vi "Teleop.vi"(10 "Match Info":T1={"Autonomous Elapsed Seconds"=0.0, "TeleOp Elapsed Seconds"=0.0, "Disabled Elapsed Seconds"=0.0, "Visited Autonomous"=FALSE, "Visited TeleOp"=FALSE, "Visited Disabled"=FALSE, "Autonomous Settings"={"Autonomous Style"=enum."Independent", "VI Refnum"=refnum}}, 11 "Call Context":T2) -> ()   [LabVIEW 2011]
doc: "This VI is called for each TeleOp packet received from the DS where the robot is not disabled. It is often used to read from the joysticks and update I/O or to update setpoints for timed control loops. It should complete and return within 20 milliseconds or it may miss DS packets."
uses:
  <vilib>/Rock Robotics/WPI/DriverStation/WPI_DriverStationDerivedRobotMode.ctl
  <vilib>/Rock Robotics/WPI/DriverStation/WPI_DriverStationMatch Info.ctl
  Robot Global Data.vi
  System Set Points and States.vi
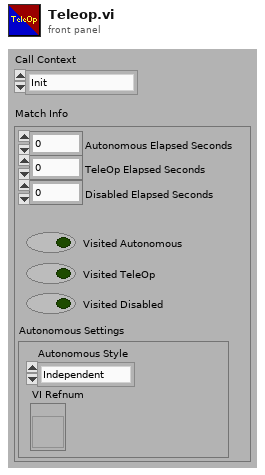
[diagram p1: front panel]
types:
  T1 = typedef "WPI_DriverStationMatch Info.ctl" = cluster{"Autonomous Elapsed Seconds":dbl, "TeleOp Elapsed Seconds":dbl, "Disabled Elapsed Seconds":dbl, "Visited Autonomous":bool, "Visited TeleOp":bool, "Visited Disabled":bool, "Autonomous Settings":cluster{"Autonomous Style":enum16{"Iterative", "Independent"}, "VI Refnum":refnum<vi>}}
  T2 = typedef "WPI_DriverStationDerivedRobotMode.ctl" = enum16{"Init", "Execute", "Stop"}
  T3 = typedef "WPI_JoystickDevRef.ctl" = cluster{"Device":T4}
  T4 = typedef "WPI_JoystickDeviceEnum.ctl" = enum16{"USB 1", "USB 2", "USB 3", "USB 4", "Kinect 1", "Kinect 2"}
  T5 = typedef "WPI_JoystickButtonState.ctl" = cluster{"Button 1":bool, "Button 2":bool, "Button 3":bool, "Button 4":bool, "Button 5":bool, "Button 6":bool, "Button 7":bool, "Button 8":bool, "Button 9":bool, "Button 10":bool, "Button 11":bool, "Button 12":bool}
  T6 = cluster{"axis 1 (x)":dbl, "axis 2 (y)":dbl, "axis 3 (throttle)":dbl, "axis 4":dbl, "axis 5":dbl, "axis 6":dbl}
  T7 = typedef "WPI_DigitalInputDevRef.ctl" = cluster{"DevStatus":errorcluster, "DIO Channel":T8, "Digital Module":T9}
  T8 = typedef "FPGA_DIOChannel.ctl" = enum8{"DIO 1", "DIO 2", "DIO 3", "DIO 4", "DIO 5", "DIO 6", "DIO 7", "DIO 8", "DIO 9", "DIO 10", "DIO 11", "DIO 12", "DIO 13", "DIO 14", "Invalid"}
  T9 = typedef "FPGA_TypedefDigitalModule.ctl" = enum16{"Digital Module 1", "Digital Module 2"}
  T10 = typedef "WPI_RobotDriveDevRef.ctl" = cluster{"DevStatus":errorcluster, "Motors[]":T11[], "Square Inputs":bool, "Max Output":dbl, "Isochronous":bool}
  T11 = typedef "WPI_MotorControlDeviceRef.ctl" = cluster{"DeviceStatus":errorcluster, "Type":enum16{"PWM", "CAN"}, "PWM":cluster{"Digital Module":T9, "PWM Channel":T12, "DeadBand":T13}, "CAN":cluster{"Device Number":u8, "Control Mode":T14, "Semaphore":T15, "Max Vout":dbl}, "Invert":bool, "TransformRef":T16, "InvTransformRef":T16}
  T12 = typedef "FPGA_DIOPWMChannel.ctl" = enum8{"PWM 1", "PWM 2", "PWM 3", "PWM 4", "PWM 5", "PWM 6", "PWM 7", "PWM 8", "PWM 9", "PWM 10", "Invalid"}
  T13 = typedef "WPI_PWMDeadband.ctl" = cluster{"Name":string, "maxPositivePwm":i32, "minPositivePwm":i32, "centerPwm":i32, "maxNegativePwm":i32, "minNegativePwm":i32, "angularRange":u16}
  T14 = typedef "WPI_CANJaguar_ControlMode.ctl" = enum8{"Percent VBus", "Current", "Speed", "Position", "Voltage"}
  T15 = typedef "Semaphore RefNum" = refnum<k1>
  T16 = typedef "WPI_PWMTransform_ConPane.ctl" = refnum<vi>
  T17 = typedef "WPI_AnalogChannelDevRef.ctl" = cluster{"DevStatus":errorcluster, "Analog Module":T18, "Analog Channel":T19}
  T18 = typedef "FPGA_TypedefAnalogModule.ctl" = enum16{"Analog Module 1", "Analog Module 2"}
  T19 = typedef "FPGA_AIChannel.ctl" = enum8{"AI 1", "AI 2", "AI 3", "AI 4", "AI 5", "AI 6", "AI 7", "AI 8", "Invalid"}
  T20 = cluster{"Position":cluster{"X":dbl, "Y":dbl}, "Distance (ft)":dbl}[]
  T21 = cluster{"Target Info[0]":cluster{"Position":cluster{"X":dbl, "Y":dbl}, "Distance (ft)":dbl}, "Target Info[1]":cluster{"Position":cluster{"X":dbl, "Y":dbl}, "Distance (ft)":dbl}, "Target Info[2]":cluster{"Position":cluster{"X":dbl, "Y":dbl}, "Distance (ft)":dbl}, "Target Info[3]":cluster{"Position":cluster{"X":dbl, "Y":dbl}, "Distance (ft)":dbl}, "Target Info[4]":cluster{"Position":cluster{"X":dbl, "Y":dbl}, "Distance (ft)":dbl}, "Target Info[5]":cluster{"Position":cluster{"X":dbl, "Y":dbl}, "Distance (ft)":dbl}, "Target Info[6]":cluster{"Position":cluster{"X":dbl, "Y":dbl}, "Distance (ft)":dbl}, "Target Info[7]":cluster{"Position":cluster{"X":dbl, "Y":dbl}, "Distance (ft)":dbl}, "Target Info[8]":cluster{"Position":cluster{"X":dbl, "Y":dbl}, "Distance (ft)":dbl}}
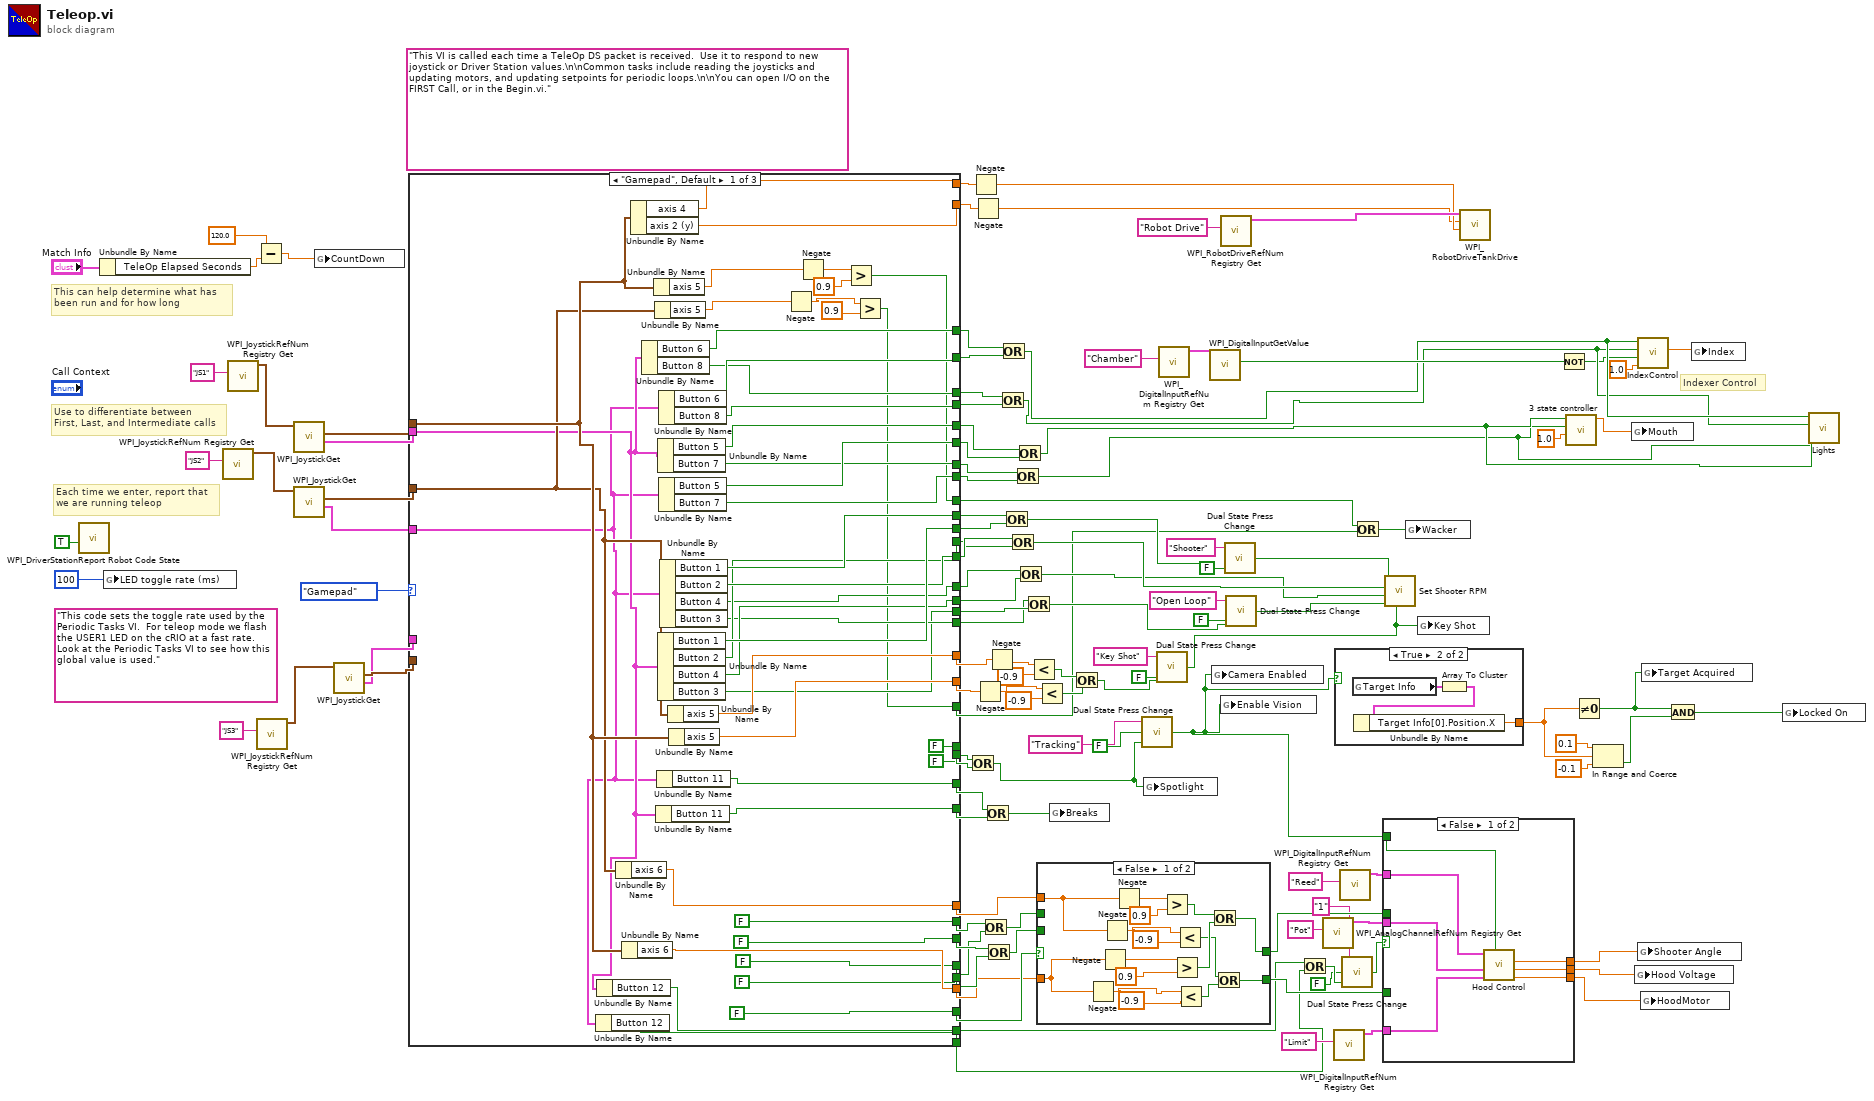
[diagram p0: block diagram]
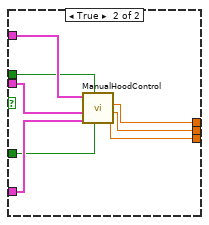
[diagram p2: hidden frame]
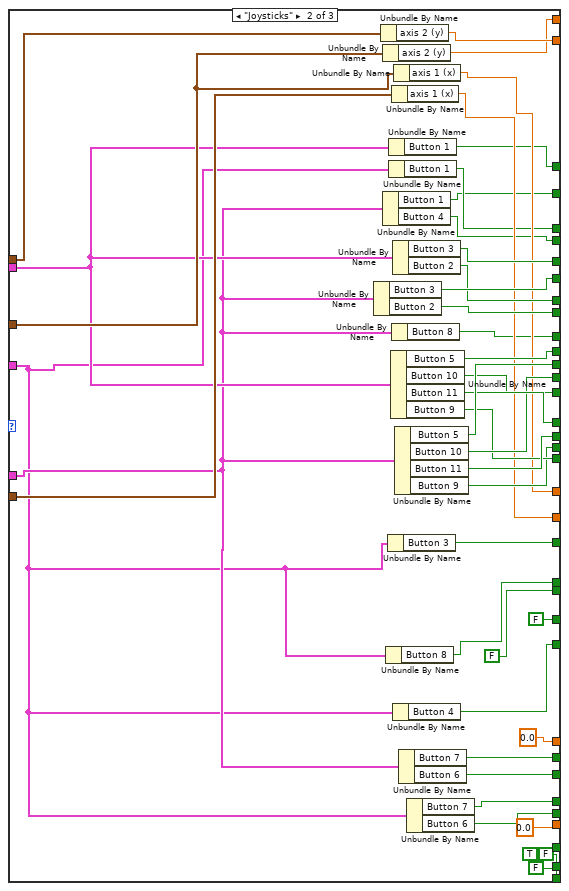
[diagram p4: hidden frame]
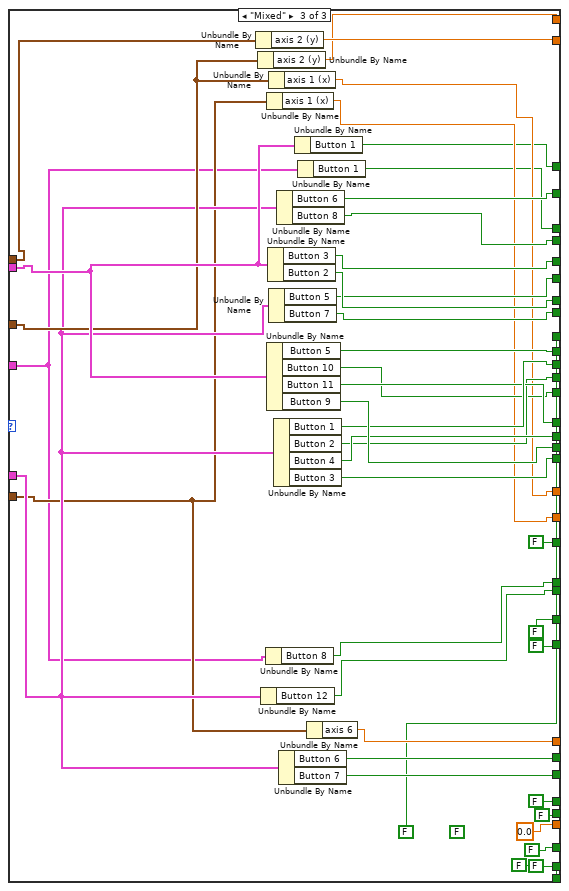
[diagram p5: hidden frame]
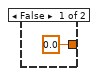
[diagram p6: hidden frame]
diagram:
  (unwired) "This code sets the toggle rate used by the Periodic Tasks VI.  For teleop mode we flash the USER1 LED on the cRIO at a fast rate.  Look at the Periodic Tasks VI to see how this global value is used."
  (unwired) "This VI is called each time a TeleOp DS packet is received.  Use it to respond to new joystick or Driver Station values.\n\nCommon tasks include reading the joysticks and updating motors, and updating setpoints for periodic loops.\n\nYou can open I/O on the FIRST Call, or in the Begin.vi."
  # "Indexer Control"
  # "Each time we enter, report that\nwe are running teleop"
  # "Use to differentiate between\nFirst, Last, and Intermediate calls"
  # "This can help determine what has\nbeen run and for how long"
  n1 = call <vilib>:"WPI_DriverStationReport Robot Code State.vi"("TeleOp"=TRUE ("Autonomous")) -> ()  [unwired: 10 in, 1 out]
  n2 = Unbundle By Name("Match Info") -> ("TeleOp Elapsed Seconds"=w94:dbl)
  n3 = global write "Robot Global Data.vi" "LED toggle rate (ms)"(u32 100 ("LED ms toggle rate")) -> ()
  n4 = call <vilib>:"WPI_JoystickRefNum Registry Get.vi"("refnum name"="JS2") -> ("JoystickDevRef"=w88:T3)  [unwired: 9 in, 1 out]
  n5 = call <vilib>:"WPI_JoystickRefNum Registry Get.vi"("refnum name"="JS1") -> ("JoystickDevRef"=w115:T3)  [unwired: 9 in, 1 out]
  n6 = Subtract(x=120.0, y=w94) -> (x-y=w60:dbl)
  n7 = call <vilib>:"WPI_JoystickRefNum Registry Get.vi"("refnum name"="JS3") -> ("JoystickDevRef"=w56:T3)  [unwired: 9 in, 1 out]
  n8 = call <vilib>:"WPI_JoystickGet.vi"("JoystickDevRef"=w115) -> ("Buttons"=w102:T5, "Axes"=w61:T6)  [unwired: 4 in, 1 out]
  n9 = call <vilib>:"WPI_JoystickGet.vi"("JoystickDevRef"=w88) -> ("Buttons"=w68:T5, "Axes"=w62:T6)  [unwired: 4 in, 1 out]
  n10 = global write "System Set Points and States.vi" "CountDown"(w60) -> ()
  n11 = call <vilib>:"WPI_JoystickGet.vi"("JoystickDevRef"=w56) -> ("Buttons"=w58:T5, "Axes"=w59:T6)  [unwired: 4 in, 1 out]
  n12 = case shown="\"Gamepad\", Default" enum16{"Gamepad", "Mixed", "Joysticks"}."Gamepad" {
    tunnel: [w164 w180 w217] -> w112
    tunnel: [w163 w181 w218] -> w111
    tunnel: w102 -> [w123 w179 w245]
    tunnel: [w162 0.0 ("axis 6") 0.0 ("axis 6")] -> w7
    tunnel: [w161 w198 w237] -> w87
    tunnel: [w160 w199 w236] -> w86
    tunnel: [w159 w196 w232] -> w84
    tunnel: [w158 w195 w233] -> w83
    tunnel: [w157 w194 w234] -> w81
    tunnel: [w156 w197 w235] -> w80
    tunnel: [w138 w192 w238] -> w78
    tunnel: [w155 w193 w239] -> w77
    tunnel: [w154 w175 w226] -> w75
    tunnel: [w153 w178 w215] -> w74
    tunnel: [w152 w177 w214] -> w72
    tunnel: [w151 w174 w227] -> w71
    tunnel: [w150 w191 w228] -> w69
    tunnel: w68 -> [w122 w169 w216]
    tunnel: [w141 w189 w230] -> w40
    tunnel: [w142 w190 w229] -> w41
    tunnel: [w149 w188 w231] -> w66
    tunnel: [FALSE ("Button 8") w200 w240] -> w64
    tunnel: [FALSE ("Button 12") FALSE ("Button 12") w222] -> w63
    tunnel: [w148 0.0 ("axis 6") w219] -> w8
    tunnel: w62 -> [w136 w182 w223]
    tunnel: w61 -> [w137 w204 w246]
    tunnel: w59 -> [_ w205 w220]
    tunnel: w58 -> [_ w173 w221]
    tunnel: [w146 w187 w225] -> w49
    tunnel: [w147 w186 w224] -> w48
    tunnel: [FALSE ("Button 6") w185 w242] -> w25
    tunnel: [FALSE ("Button 7") w184 w241] -> w29
    tunnel: [FALSE TRUE FALSE] -> w47
    tunnel: [w129 w176 FALSE ("Button 1")] -> w31
    tunnel: [w128 w172 FALSE ("Button 3")] -> w32
    tunnel: [FALSE ("Button 7") w171 FALSE ("Button 7")] -> w28
    tunnel: [FALSE ("Button 6") w170 FALSE ("Button 6")] -> w26
    tunnel: [w125 FALSE ("Button 12") FALSE ("Button 4")] -> w19
    tunnel: [w124 w168 FALSE ("Button 4")] -> w18
    tunnel: [w121 FALSE ("Button 11") FALSE ("Button 11")] -> w2
    tunnel: [w120 FALSE ("Button 11") FALSE ("Button 11")] -> w1
    frame "Gamepad", Default {
      n13 = Unbundle By Name(w122) -> ("Button 12"=w120:bool)
      n14 = Unbundle By Name(w123) -> ("Button 12"=w121:bool)
      n15 = Unbundle By Name(w136) -> ("axis 6"=w148:dbl)
      n16 = Unbundle By Name(w137) -> ("axis 6"=w162:dbl)
      n17 = Unbundle By Name(w137) -> ("axis 4"=w164:dbl, "axis 2 (y)"=w163:dbl)
      n18 = Unbundle By Name(w123) -> ("Button 6"=w153:bool, "Button 8"=w152:bool)
      n19 = Unbundle By Name(w137) -> ("axis 5"=w135:dbl)
      n20 = Unbundle By Name(w136) -> ("axis 5"=w134:dbl)
      n21 = Unbundle By Name(w123) -> ("Button 11"=w124:bool)
      n22 = Unbundle By Name(w122) -> ("Button 11"=w125:bool)
      n23 = Unbundle By Name(w123) -> ("Button 5"=w150:bool, "Button 7"=w141:bool)
      n24 = Unbundle By Name(w123) -> ("Button 1"=w160:bool, "Button 2"=w158:bool, "Button 4"=w157:bool, "Button 3"=w138:bool)
      n25 = Unbundle By Name(w122) -> ("Button 6"=w154:bool, "Button 8"=w151:bool)
      n26 = Unbundle By Name(w122) -> ("Button 5"=w142:bool, "Button 7"=w149:bool)
      n27 = Unbundle By Name(w122) -> ("Button 1"=w161:bool, "Button 2"=w159:bool, "Button 4"=w156:bool, "Button 3"=w155:bool)
      n28 = Unbundle By Name(w136) -> ("axis 5"=w147:dbl)
      n29 = Unbundle By Name(w137) -> ("axis 5"=w146:dbl)
      n30 = Negate(x=w134) -> (-x=w131:dbl)
      n31 = Negate(x=w135) -> (-x=w133:dbl)
      n32 = Greater?(x=w133, y=0.9) -> (0:w129:bool)
      n33 = Greater?(x=w131, y=0.9) -> (0:w128:bool)
    }
    frame "Joysticks" {
      n34 = Unbundle By Name(w173) -> ("Button 3"=w190:bool, "Button 2"=w188:bool)
      n35 = Unbundle By Name(w204) -> ("axis 2 (y)"=w181:dbl)
      n36 = Unbundle By Name(w182) -> ("axis 2 (y)"=w180:dbl)
      n37 = Unbundle By Name(w173) -> ("Button 1"=w175:bool, "Button 4"=w174:bool)
      n38 = Unbundle By Name(w169) -> ("Button 8"=w200:bool)
      n39 = Unbundle By Name(w169) -> ("Button 3"=w172:bool)
      n40 = Unbundle By Name(w179) -> ("Button 1"=w178:bool)
      n41 = Unbundle By Name(w169) -> ("Button 1"=w177:bool)
      n42 = Unbundle By Name(w179) -> ("Button 5"=w198:bool, "Button 10"=w196:bool, "Button 11"=w197:bool, "Button 9"=w193:bool)
      n43 = Unbundle By Name(w205) -> ("axis 1 (x)"=w187:dbl)
      n44 = Unbundle By Name(w173) -> ("Button 8"=w176:bool)
      n45 = Unbundle By Name(w179) -> ("Button 3"=w191:bool, "Button 2"=w189:bool)
      n46 = Unbundle By Name(w169) -> ("Button 4"=w168:bool)
      n47 = Unbundle By Name(w182) -> ("axis 1 (x)"=w186:dbl)
      n48 = Unbundle By Name(w173) -> ("Button 5"=w199:bool, "Button 10"=w195:bool, "Button 11"=w194:bool, "Button 9"=w192:bool)
      n49 = Unbundle By Name(w173) -> ("Button 7"=w185:bool, "Button 6"=w184:bool)
      n50 = Unbundle By Name(w169) -> ("Button 7"=w170:bool, "Button 6"=w171:bool)
    }
    frame "Mixed" {
      (unwired) FALSE ("Button 4")
      n51 = Unbundle By Name(w246) -> ("axis 2 (y)"=w218:dbl)
      n52 = Unbundle By Name(w223) -> ("axis 2 (y)"=w217:dbl)
      n53 = Unbundle By Name(w221) -> ("Button 12"=w222:bool)
      n54 = Unbundle By Name(w216) -> ("Button 8"=w240:bool)
      n55 = Unbundle By Name(w220) -> ("axis 1 (x)"=w225:dbl)
      n56 = Unbundle By Name(w245) -> ("Button 5"=w237:bool, "Button 10"=w232:bool, "Button 11"=w235:bool, "Button 9"=w238:bool)
      n57 = Unbundle By Name(w245) -> ("Button 3"=w228:bool, "Button 2"=w230:bool)
      n58 = Unbundle By Name(w223) -> ("axis 1 (x)"=w224:dbl)
      n59 = Unbundle By Name(w221) -> ("Button 5"=w229:bool, "Button 7"=w231:bool)
      n60 = Unbundle By Name(w221) -> ("Button 1"=w236:bool, "Button 2"=w233:bool, "Button 4"=w234:bool, "Button 3"=w239:bool)
      n61 = Unbundle By Name(w221) -> ("Button 6"=w226:bool, "Button 8"=w227:bool)
      n62 = Unbundle By Name(w221) -> ("Button 6"=w242:bool, "Button 7"=w241:bool)
      n63 = Unbundle By Name(w245) -> ("Button 1"=w215:bool)
      n64 = Unbundle By Name(w216) -> ("Button 1"=w214:bool)
      n65 = Unbundle By Name(w220) -> ("axis 6"=w219:dbl)
    }
  }
  n66 = Or(x=w64, y=w63) -> (x .or. y?=w37:bool)
  n67 = Negate(x=w112) -> (-x=w43:dbl)
  n68 = Negate(x=w111) -> (-x=w42:dbl)
  n69 = Negate(x=w49) -> (-x=w52:dbl)
  n70 = Or(x=w25, y=w26) -> (x .or. y?=w27:bool)
  n71 = Or(x=w19, y=w18) -> (x .or. y?=w20:bool)
  n72 = Or(x=w29, y=w28) -> (x .or. y?=w30:bool)
  n73 = Negate(x=w48) -> (-x=w54:dbl)
  n74 = Or(x=w72, y=w71) -> (x .or. y?=w70:bool)
  n75 = Or(x=w74, y=w75) -> (x .or. y?=w73:bool)
  n76 = Or(x=w87, y=w86) -> (x .or. y?=w85:bool)
  n77 = Or(x=w84, y=w83) -> (x .or. y?=w82:bool)
  n78 = Or(x=w40, y=w66) -> (x .or. y?=w65:bool)
  n79 = Or(x=w69, y=w41) -> (x .or. y?=w67:bool)
  n80 = Or(x=w80, y=w81) -> (x .or. y?=w79:bool)
  n81 = Or(x=w77, y=w78) -> (x .or. y?=w76:bool)
  n82 = Less?(x=w54, y=-0.9) -> (x < y?=w51:bool)
  n83 = Less?(x=w52, y=-0.9) -> (x < y?=w50:bool)
  n84 = case shown="False" w47 {
    tunnel: w7 -> [w253 _]
    tunnel: w8 -> [w254 _]
    tunnel: [w250 w263] -> w10
    tunnel: [w247 w264] -> w9
    tunnel: w27 -> [_ w264]
    tunnel: w30 -> [_ w263]
    frame False {
      n85 = Negate(x=w253) -> (-x=w258:dbl)
      n86 = Negate(x=w253) -> (-x=w260:dbl)
      n87 = Negate(x=w254) -> (-x=w255:dbl)
      n88 = Negate(x=w254) -> (-x=w262:dbl)
      n89 = Greater?(x=w262, y=0.9) -> (0:w252:bool)
      n90 = Greater?(x=w260, y=0.9) -> (0:w251:bool)
      n91 = Less?(x=w255, y=-0.9) -> (x < y?=w249:bool)
      n92 = Less?(x=w258, y=-0.9) -> (x < y?=w248:bool)
      n93 = Or(x=w252, y=w251) -> (x .or. y?=w250:bool)
      n94 = Or(x=w249, y=w248) -> (x .or. y?=w247:bool)
    }
    frame True {
    }
  }
  n95 = global write "System Set Points and States.vi" "Breaks"(w20) -> ()
  n96 = Or(x=w51, y=w50) -> (x .or. y?=w44:bool)
  n97 = call "Dual State Press Change.vi"("Enable/Disable"=w37, "Initial"=FALSE, "Value Name"="Tracking") -> ("Enabled"=w92:bool)
  n98 = global write "System Set Points and States.vi" "Spotlight"(w37) -> ()
  n99 = call "Dual State Press Change.vi"("Enable/Disable"=w44, "Initial"=FALSE, "Value Name"="Key Shot") -> ("Enabled"=w17:bool)
  n100 = call <vilib>:"WPI_DigitalInputRefNum Registry Get.vi"("refnum name"="Chamber") -> ("DigitalInputDevRef"=w110:T7)  [unwired: 9 in, 1 out]
  n101 = call <vilib>:"WPI_DigitalInputGetValue.vi"("DigitalInputDevRef"=w110) -> ("Value"=w108:bool)  [unwired: 8 in, 2 out]
  n102 = global write "System Set Points and States.vi" "Camera Enabled"(w92) -> ()
  n103 = call <vilib>:"WPI_RobotDriveRefNum Registry Get.vi"("refnum name"="Robot Drive") -> ("RobotDriveDevRef"=w113:T10)  [unwired: 9 in, 1 out]
  n104 = global write "Robot Global Data.vi" "Enable Vision"(w92) -> ()
  n105 = call "Dual State Press Change.vi"("Enable/Disable"=w85, "Initial"=FALSE, "Value Name"="Shooter") -> ("Enabled"=w38:bool)
  n106 = call "Dual State Press Change.vi"("Enable/Disable"=w76, "Initial"=FALSE, "Value Name"="Open Loop") -> ("Enabled"=w103:bool)
  n107 = Or(x=w2, y=w1) -> (x .or. y?=w6:bool)
  n108 = call <vilib>:"WPI_AnalogChannelRefNum Registry Get.vi"("refnum name"="Pot") -> ("AIDeviceRef"=w11:T17)  [unwired: 9 in, 1 out]
  n109 = call <vilib>:"WPI_DigitalInputRefNum Registry Get.vi"("refnum name"="Limit") -> ("DigitalInputDevRef"=w13:T7)  [unwired: 9 in, 1 out]
  n110 = case shown="True" w92 {
    tunnel: [0.0 ("Distance (ft)") w266] -> w95
    frame False {
    }
    frame True {
      n111 = global read "Robot Global Data.vi" "Target Info"() -> (w268:T20)
      n112 = Array To Cluster(array=w268) -> (cluster=w267:T21)
      n113 = Unbundle By Name(w267) -> ("Target Info[0].Position.X"=w266:dbl)
    }
  }
  n114 = call <vilib>:"WPI_DigitalInputRefNum Registry Get.vi"("refnum name"="Reed") -> ("DigitalInputDevRef"=w14:T7)  [unwired: 9 in, 1 out]
  n115 = call "Dual State Press Change.vi"("Enable/Disable"=w6, "Initial"=FALSE, "Value Name"="1") -> ("Enabled"=w3:bool)
  n116 = Or(x=w31, y=w32) -> (x .or. y?=w24:bool)
  n117 = case shown="False" w3 {
    tunnel: w92 -> [w275 _]
    tunnel: [w274 w278] -> w91
    tunnel: [w273 w277] -> w90
    tunnel: [w272 w276] -> w21
    tunnel: w14 -> [w271 w282]
    tunnel: w13 -> [w270 w283]
    tunnel: w11 -> [w269 w281]
    tunnel: w10 -> [_ w280]
    tunnel: w9 -> [_ w279]
    frame False {
      n118 = call "Hood Control.vi"("Vision"=w275, "Top"=w270, "AIDeviceRef"=w269, "Bottom"=w271) -> ("HoodSpeed"=w272:dbl, "Voltage"=w273:dbl, "Shoter Angle"=w274:dbl)  [unwired: 5 in]
    }
    frame True {
      n119 = call "ManualHoodControl.vi"("Down"=w279, "Up"=w280, "Top"=w283, "AIDeviceRef"=w281, "Bottom"=w282) -> ("Hood Speed"=w276:dbl, "Voltage"=w277:dbl, "Shoter Angle"=w278:dbl)  [unwired: 4 in]
    }
  }
  n120 = call "Set Shooter RPM.vi"("Key Shot"=w17, "Open Loop"=w103, "Increment"=w79, "Decrement"=w82, "Shooter Enabled"=w38) -> ()  [unwired: 7 in]
  n121 = global write "System Set Points and States.vi" "Wacker"(w24) -> ()
  n122 = global write "System Set Points and States.vi" "Key Shot"(w17) -> ()
  n123 = call <vilib>:"WPI_RobotDriveTankDrive.vi"("Right axis value"=w43, "Left axis value"=w42, "RobotDriveDevRef"=w113) -> ()  [unwired: 7 in, 2 out]
  n124 = Not(x=w108) -> (.not. x?=w34:bool)
  n125 = call "3 state controller.vi"("Power"=1.0, "Backward"=w65, "Forward"=w67) -> ("Numeric"=w23:dbl)  [unwired: 8 in]
  n126 = Not Equal To 0?(x=w95) -> (x != 0?=w33:bool)
  n127 = In Range and Coerce(upper limit=0.1, x=w95, lower limit=-0.1) -> (In Range?=w97:bool)  [unwired: 1 out]
  n128 = global write "System Set Points and States.vi" "Mouth"(w23) -> ()
  n129 = global write "System Set Points and States.vi" "Hood Voltage"(w90) -> ()
  n130 = call "IndexControl.vi"("Power"=1.0, "Chamber"=w34, "Back"=w70, "Forward"=w73) -> ("Numeric"=w22:dbl)  [unwired: 7 in]
  n131 = global write "System Set Points and States.vi" "Shooter Angle"(w91) -> ()
  n132 = global write "System Set Points and States.vi" "HoodMotor"(w21) -> ()
  n133 = global write "System Set Points and States.vi" "Target Acquired"(w33) -> ()
  n134 = And(x=w33, y=w97) -> (x .and. y?=w96:bool)
  n135 = global write "System Set Points and States.vi" "Index"(w22) -> ()
  n136 = global write "System Set Points and States.vi" "Locked On"(w96) -> ()
  n137 = call "Lights.vi"("Input4"=w67, "Input3"=w65, "Input2"=w70, "Input1"=w73) -> ()  [unwired: 8 in]
